vi "Frames verwerten.vi"(10 "CAN Messdaten":T3, 11 "Konfig Daten":T1={"Baude Rate"=250000, "COM state"=0, "Frame-ID FTIR Start"=0, "Frame-ID FTIR End"=0, "Frame-ID Status Start"=0, "Frame-ID Status End"=0, "Zustand Information"=0, "Aktion"=0, "Frame-ID FTIR Arry"=[], "Frame-ID Status Arry"=[], "GPS Start"=0, "Interface"="CAN1"} {"Baude Rate" items=["40 kBaud"=40000, "50 kBaud"=50000, "62,5 kBaud"=62500, "80 kBaud"=80000, "83,3 kBaud"=83300, "100 kBaud"=100000, "125 kBaud"=125000, "160 kBaud"=160000, "200 kBaud"=200000, "250 kBaud"=250000, "400 kBaud"=400000, "500 kBaud"=500000, "800 kBaud"=800000, "1 MBaud"=1000000]}) -> (3 "Ausgangs-Cluster":T1={"Baude Rate"=250000, "COM state"=0, "Frame-ID FTIR Start"=0, "Frame-ID FTIR End"=0, "Frame-ID Status Start"=0, "Frame-ID Status End"=0, "Zustand Information"=0, "Aktion"=0, "Frame-ID FTIR Arry"=[], "Frame-ID Status Arry"=[], "GPS Start"=0, "Interface"="CAN1"} {"Baude Rate" items=["40 kBaud"=40000, "50 kBaud"=50000, "62,5 kBaud"=62500, "80 kBaud"=80000, "83,3 kBaud"=83300, "100 kBaud"=100000, "125 kBaud"=125000, "160 kBaud"=160000, "200 kBaud"=200000, "250 kBaud"=250000, "400 kBaud"=400000, "500 kBaud"=500000, "800 kBaud"=800000, "1 MBaud"=1000000]})   [LabVIEW 2020, in "CAN Konfig.lvlib"]
uses:
  CAN Konfig.lvlib
  Konfig Daten PC.ctl
  cRIO/CAN Interface/Baude Rate.ctl
  CAN Messdaten.ctl
  Aktion FGV CAN.ctl
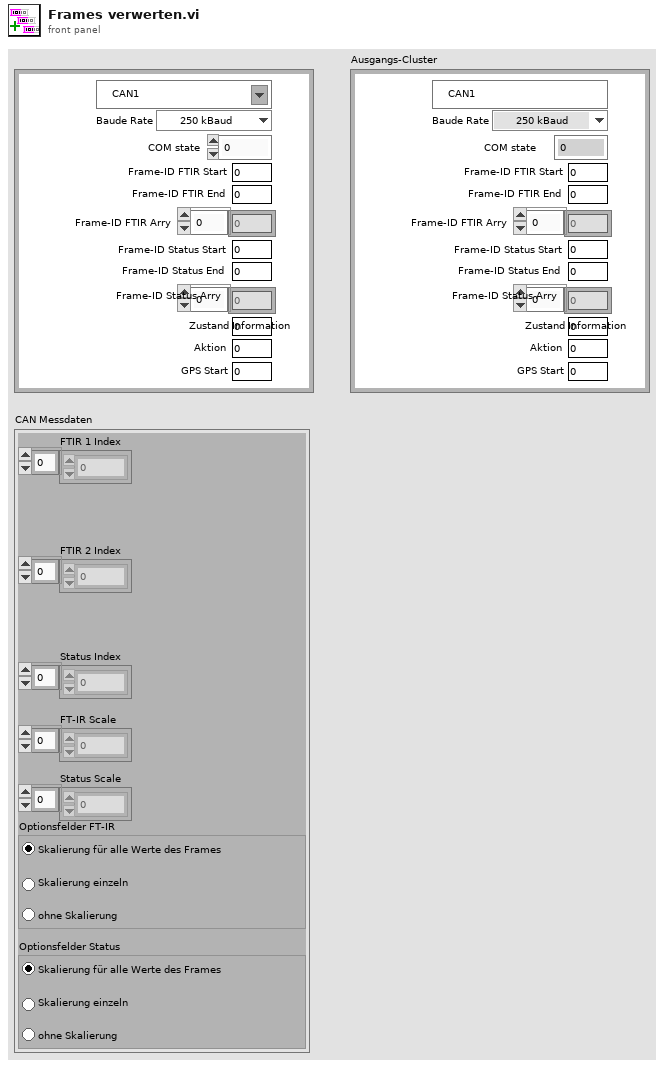
[diagram p1: front panel]
types:
  T1 = typedef "CAN Konfig.lvlib/Konfig Daten PC.ctl" = cluster{"Baude Rate":T2, "COM state":u8, "Frame-ID FTIR Start":u32, "Frame-ID FTIR End":u32, "Frame-ID Status Start":u32, "Frame-ID Status End":u32, "Zustand Information":u32, "Aktion":u32, "Frame-ID FTIR Arry":u32[], "Frame-ID Status Arry":u32[], "GPS Start":u32, "Interface":refnum<k21>}
  T2 = typedef "CAN Interface.lvlib/Baude Rate.ctl" = u32
  T3 = typedef "CAN Konfig.lvlib/CAN Messdaten.ctl" = cluster{"FTIR 1 Index":i32[], "FTIR 2 Index":i32[], "Status Index":i32[], "FT-IR Scale":sgl[], "Status Scale":sgl[], "Optionsfelder FT-IR":enum32{"Optionsauswahl 1", "Optionsauswahl 2", "Optionsauswahl 3"}, "Optionsfelder Status":enum32{"Optionsauswahl 1", "Optionsauswahl 2", "Optionsauswahl 3"}}
  T4 = typedef "CAN Konfig.lvlib/Aktion FGV CAN.ctl" = enum16{"lesen", "schreiben Konfig", "Status", "Messdaten", "laden", "speichern", "CAN Data"}
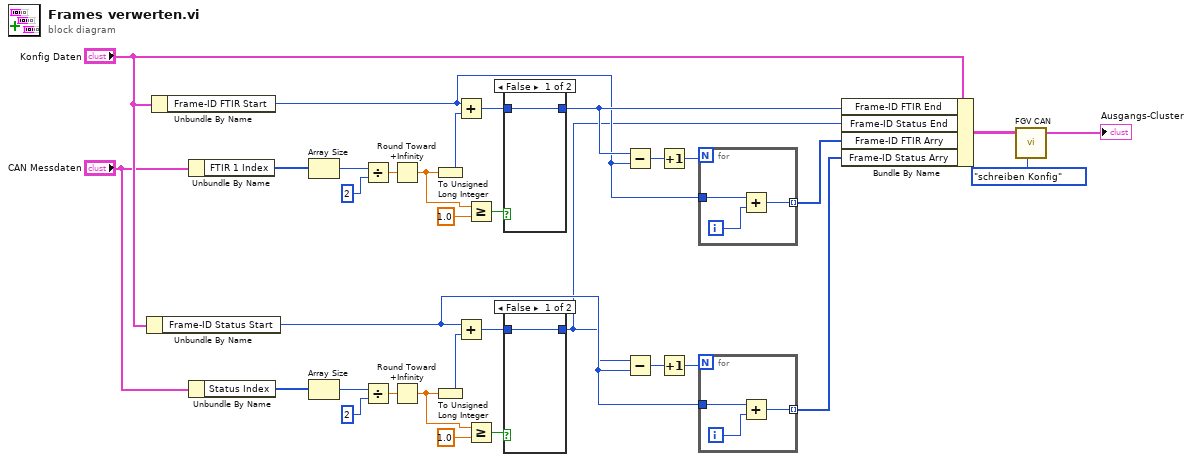
[diagram p0: block diagram]
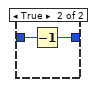
[diagram p2: hidden frame]
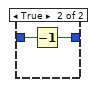
[diagram p3: hidden frame]
diagram:
  n1 = Unbundle By Name("Konfig Daten") -> ("Frame-ID Status Start"=w3:u32)
  n2 = Unbundle By Name("Konfig Daten") -> ("Frame-ID FTIR Start"=w9:u32)
  n3 = Unbundle By Name("CAN Messdaten") -> ("FTIR 1 Index"=w31:i32[])
  n4 = Unbundle By Name("CAN Messdaten") -> ("Status Index"=w13:i32[])
  n5 = Array Size(array=w31) -> (size(s)=w30:i32)
  n6 = Array Size(array=w13) -> (size(s)=w14:i32)
  n7 = Divide(x=w30, y=2) -> (x/y=w24:dbl)
  n8 = Divide(x=w14, y=2) -> (x/y=w19:dbl)
  n9 = Round Toward +Infinity(x=w24) -> (ceil(x): smallest int >= x=w23:dbl)
  n10 = Round Toward +Infinity(x=w19) -> (ceil(x): smallest int >= x=w20:dbl)
  n11 = To Unsigned Long Integer(number=w23) -> (unsigned 32bit integer=w28:u32)
  n12 = To Unsigned Long Integer(number=w20) -> (unsigned 32bit integer=w16:u32)
  n13 = Add(x=w9, y=w28) -> (x+y=w27:u32)
  n14 = Add(x=w3, y=w16) -> (x+y=w17:u32)
  n15 = Greater Or Equal?(x=w23, y=1.0) -> (x >= y?=w25:bool)
  n16 = Greater Or Equal?(x=w20, y=1.0) -> (x >= y?=w18:bool)
  n17 = case shown="False" w25 {
    tunnel: w27 -> [w33 w35]
    tunnel: [w33 w34] -> w10
    frame False {
    }
    frame True {
      n18 = Decrement(x=w35) -> (x-1=w34:u32)
    }
  }
  n19 = case shown="False" w18 {
    tunnel: w17 -> [w36 w38]
    tunnel: [w36 w37] -> w2
    frame False {
    }
    frame True {
      n20 = Decrement(x=w38) -> (x-1=w37:u32)
    }
  }
  n21 = Subtract(x=w10, y=w9) -> (x-y=w8:u32)
  n22 = Subtract(x=w2, y=w3) -> (x-y=w4:u32)
  n23 = Increment(x=w8) -> (x+1=w7:u32)
  n24 = Increment(x=w4) -> (x+1=w5:u32)
  n25 = for {
    N: w7 -> [_]
    tunnel: w9 -> [w41]
    tunnel: [w40] -> w6 mode=indexing
    i -> [w39]
    n26 = Add(x=w41, y=w39) -> (x+y=w40:u32)
  }
  n27 = for {
    N: w5 -> [_]
    tunnel: w3 -> [w44]
    tunnel: [w43] -> w1 mode=indexing
    i -> [w42]
    n28 = Add(x=w44, y=w42) -> (x+y=w43:u32)
  }
  n29 = Bundle By Name(cluster="Konfig Daten", "Frame-ID FTIR End"=w10, "Frame-ID Status End"=w2, "Frame-ID FTIR Arry"=w6, "Frame-ID Status Arry"=w1) -> (w26:T1)
  "Ausgangs-Cluster" <- w26
  n30 = call "FGV CAN.vi"("Aktion"=Aktion_FGV_CAN."schreiben Konfig", "Konfig Daten"=w26) -> ()  [unwired: 5 in, 5 out]
